vi "excel测试.vi"() -> ()   [LabVIEW 2015]
panel:
  in  "操作者":string
  in  "实验地点":string
  out "短轴半径":string[](array[string])
  out "长轴半径":string[](array[string])
  out "长轴原曲线":dbl[](graph)
  out "短轴原曲线":dbl[](graph)
  out "周长":dbl
  out "短轴M2因子":dbl
  out "位置":string[](array[string])
  out "质心坐标X":dbl
  out "质心坐标Y":dbl
  out "面积":dbl
  out "短轴拟合曲线":dbl[](graph)
  out "长轴M2因子":dbl
  out "长轴拟合曲线":dbl[](graph)
  out "横轴拟合曲线":dbl[](graph)
  out "横轴原曲线":dbl[](graph)
  out "纵轴原曲线":dbl[](graph)
  out "纵轴拟合曲线":dbl[](graph)
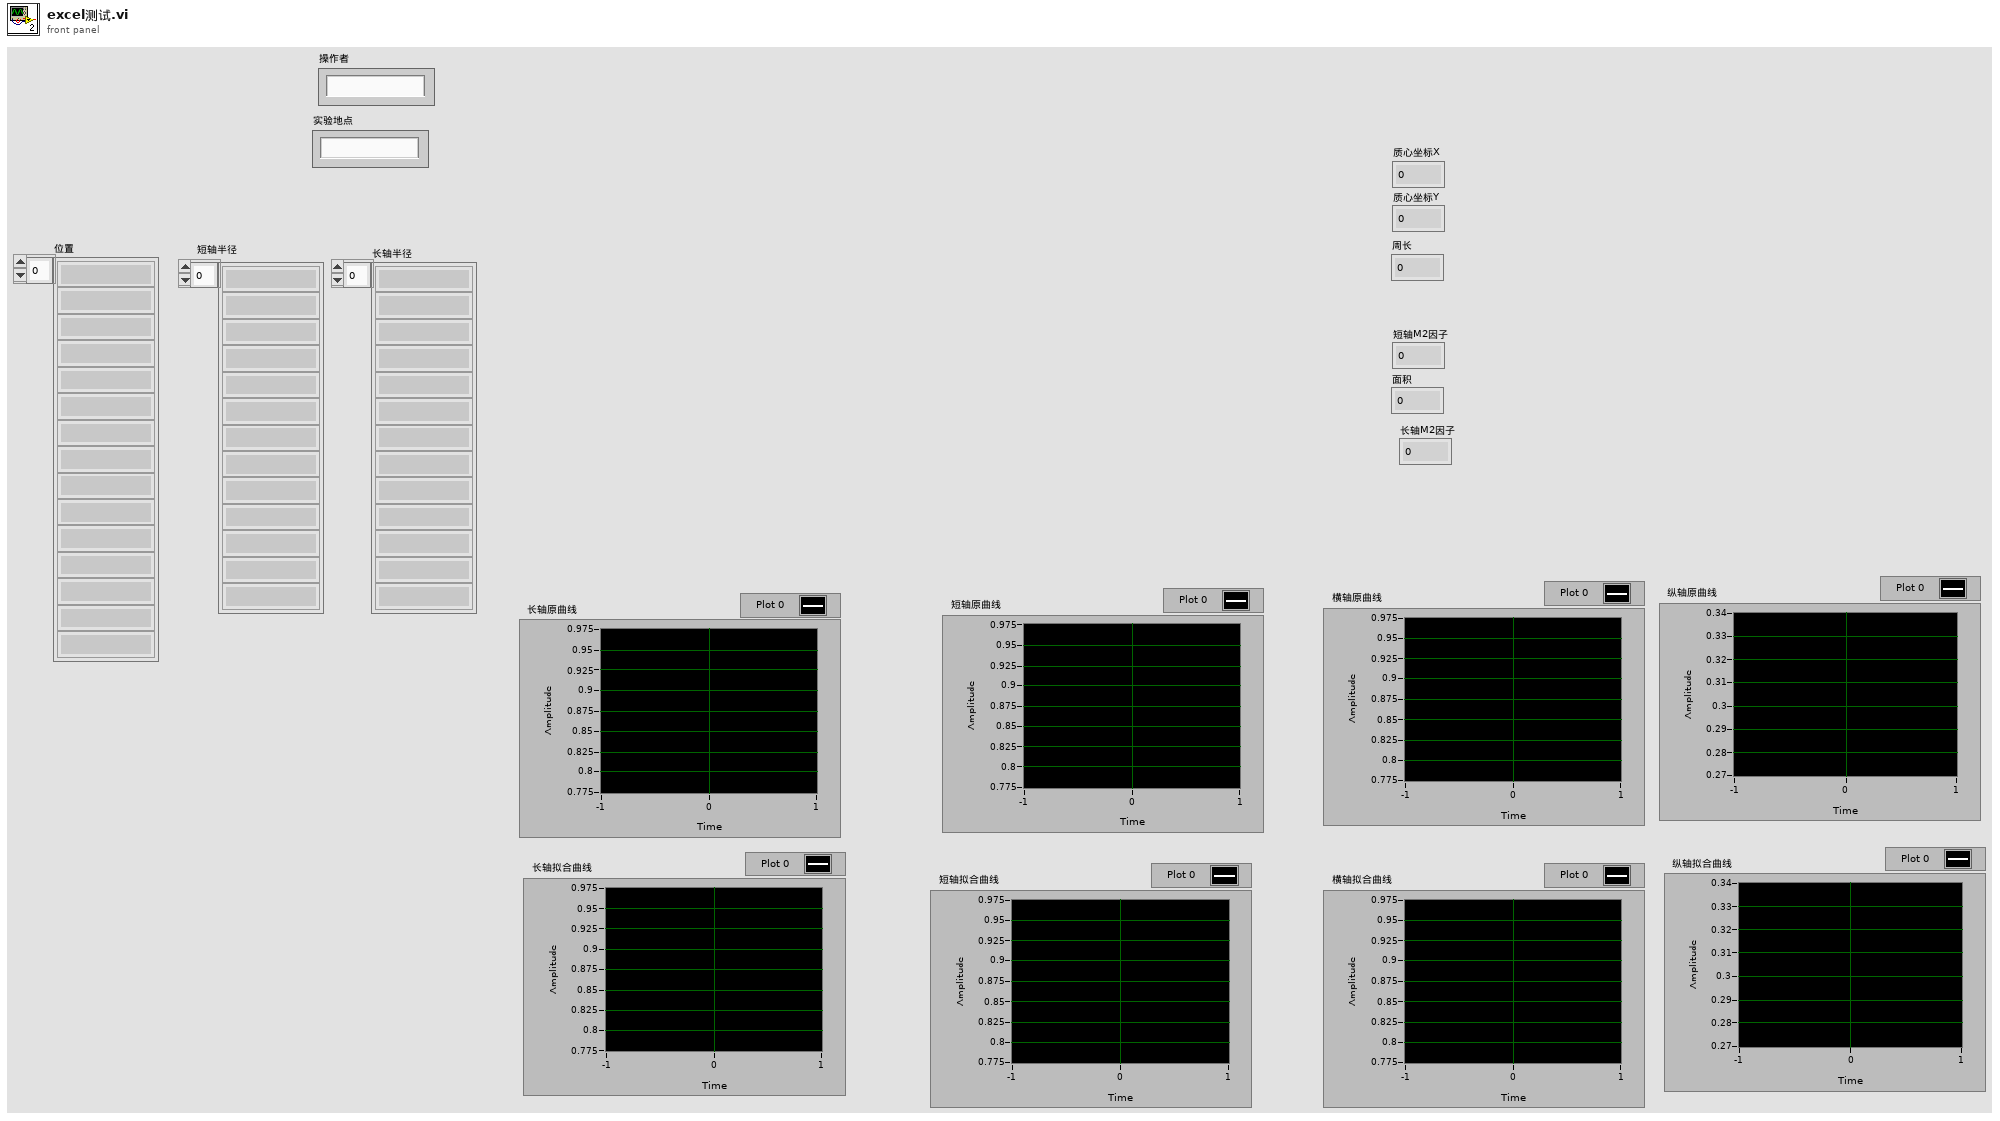
[diagram p1: front panel]
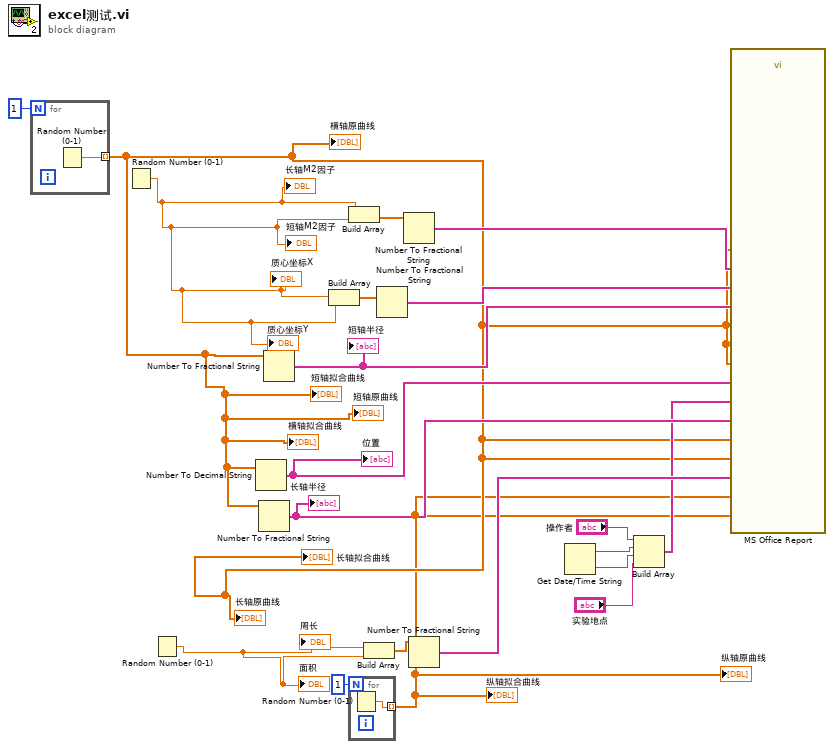
[diagram p0: block diagram]
diagram:
  n1 = for {
    N: 1 -> [_]
    tunnel: [w21] -> w4 mode=indexing
    n2 = Random Number (0-1)() -> (number: 0 to 1=w21:dbl)
  }
  "长轴原曲线" <- w4
  "短轴原曲线" <- w4
  "短轴拟合曲线" <- w4
  "长轴拟合曲线" <- w4
  "横轴拟合曲线" <- w4
  "横轴原曲线" <- w4
  n3 = Random Number (0-1)() -> (number: 0 to 1=w5:dbl)
  "短轴M2因子" <- w5
  "质心坐标X" <- w5
  "质心坐标Y" <- w5
  "长轴M2因子" <- w5
  n4 = Random Number (0-1)() -> (number: 0 to 1=w3:dbl)
  "周长" <- w3
  "面积" <- w3
  n5 = Number To Decimal String(number=w4) -> (decimal integer string=w15:string[])  [unwired: 1 in]
  "位置" <- w15
  n6 = Number To Fractional String(number=w4) -> (F-format string=w14:string[])  [unwired: 3 in]
  "长轴半径" <- w14
  n7 = Number To Fractional String(number=w4) -> (F-format string=w16:string[])  [unwired: 3 in]
  "短轴半径" <- w16
  n8 = Build Array(w5, w5) -> (w18:dbl[])
  n9 = Build Array(w5, w5) -> (w20:dbl[])
  n10 = for {
    N: 1 -> [_]
    tunnel: [w22] -> w1 mode=indexing
    n11 = Random Number (0-1)() -> (number: 0 to 1=w22:dbl)
  }
  "纵轴原曲线" <- w1
  "纵轴拟合曲线" <- w1
  n12 = Build Array(w3, w3) -> (w13:dbl[])
  n13 = Number To Fractional String(number=w18) -> (F-format string=w17:string[])  [unwired: 3 in]
  n14 = Number To Fractional String(number=w20) -> (F-format string=w19:string[])  [unwired: 3 in]
  n15 = Number To Fractional String(number=w13) -> (F-format string=w12:string[])  [unwired: 3 in]
  n16 = Get Date/Time String() -> (date string=w10:string, time string=w9:string)  [unwired: 3 in]
  n17 = Build Array("操作者", w10, w9, "实验地点") -> (w7:string[])
  n18 = call "MS Office Report"("M2因子"=w19, "XY"=w17, "短轴半径"=w16, "短轴拟合曲线"=w4, "短轴原曲线"=w4, "横轴拟合曲线"=w4, "横轴原曲线"=w4, "位置"=w15, "信息"=w7, "长轴半径"=w14, "长轴拟合曲线"=w4, "长轴原曲线"=w4, "周长与面积"=w12, "纵轴拟合曲线"=w1, "纵轴原曲线"=w1) -> ()  [unwired: 12 in, 1 out]
